vi "aFGV - Read Write Config.vi"(6 "State":enum16{"Read", "Write", "Delete"}(ring), 7 "Section":T1=enum."Calibration", 8 "Error In":errorcluster, 10 "Key Name":string, 11 "Data in":string[](array[string])) -> (0 "Error Out":errorcluster, 2 "Data out":string[](array[string]), 3 "Key Names":string[](array[string]))   [LabVIEW 2020]
uses:
  Control/Section.ctl
  Control/State - FGV.ctl
  <vilib>/Utility/config.llb/Read Key (String).vi
  <vilib>/Utility/config.llb/Write Key (String).vi
  <vilib>/Utility/config.llb/NI_LVConfig.lvlib
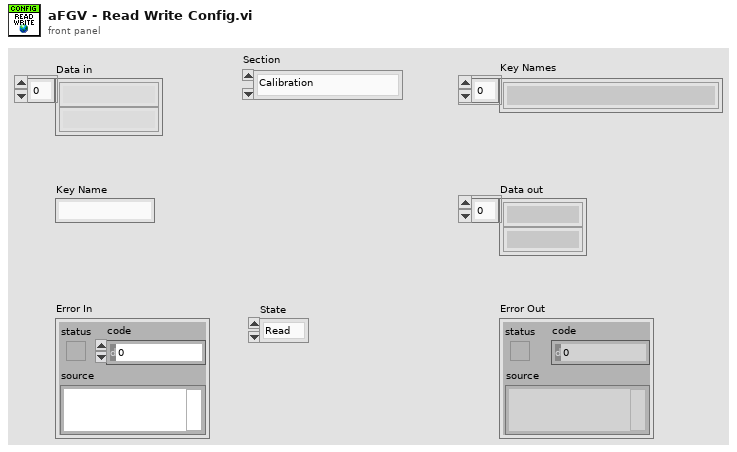
[diagram p1: front panel]
types:
  T1 = typedef "Section.ctl" = enum16{"Software Setup", "Config", "Setup", "Network Stream", "MQTT Client", "Setting", "Sample Interval", "Calibration", "Pre-Ranging", "Overrun", "Static", "Filter", "Properties", "Alarm", "Device", "Logging"}
  T2 = typedef "State - FGV.ctl" = enum16{"Write", "Read"}
  T3 = typedef "NI_LVConfig.lvlib/Config Data RefNum.ctl" = refnum<k1>
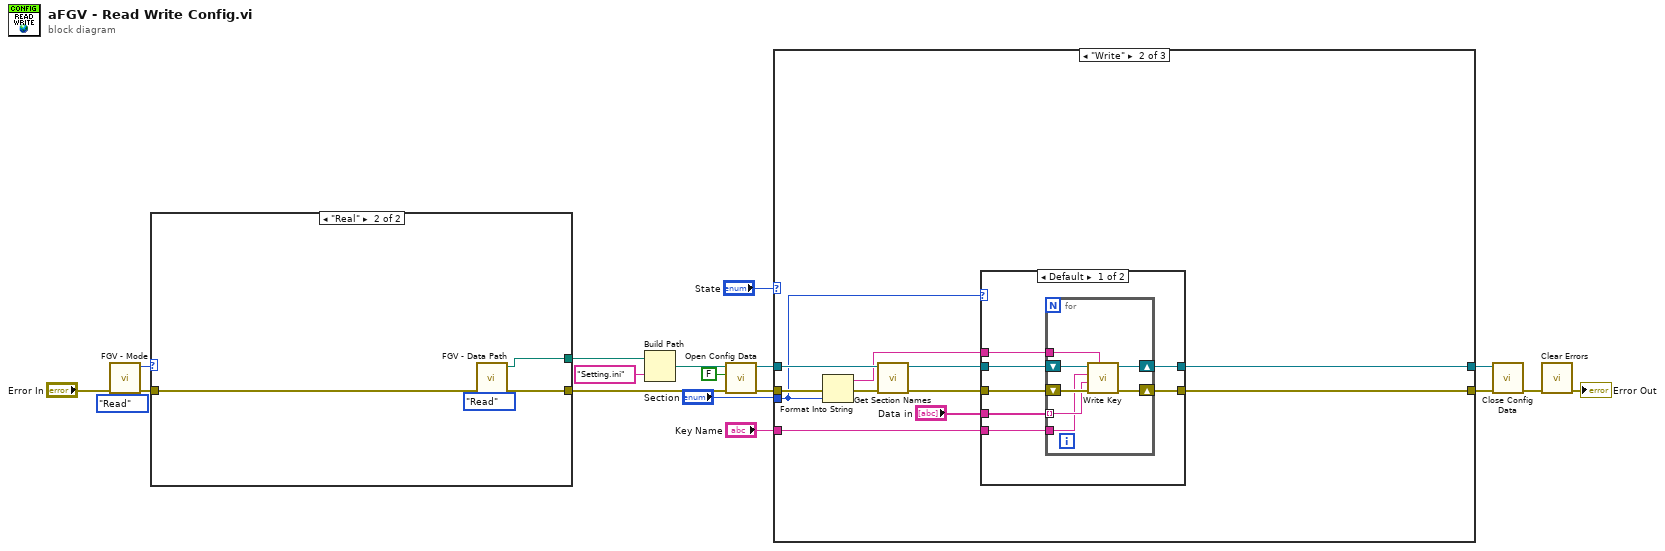
[diagram p0: block diagram]
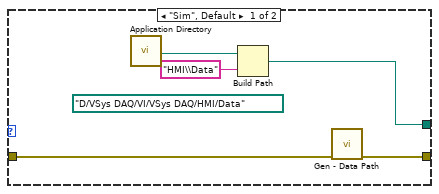
[diagram p2: hidden frame]
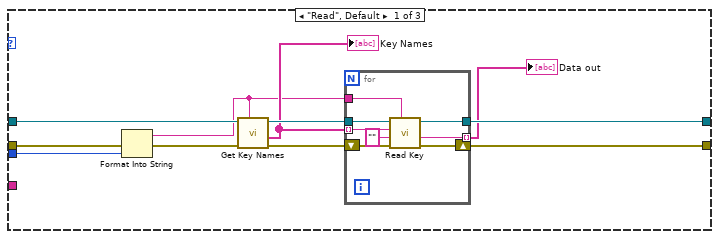
[diagram p3: hidden frame]
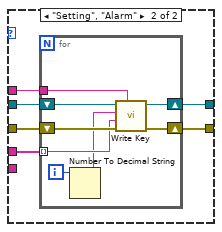
[diagram p4: hidden frame]
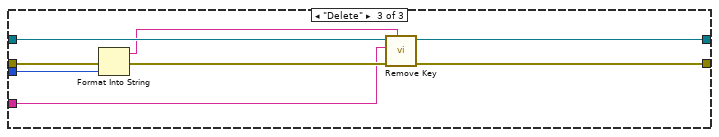
[diagram p5: hidden frame]
diagram:
  n1 = call "FGV - Mode.vi"("Action"=enum16{"Read", "Write"}."Read", "Error In"="Error In") -> ("Error Out"=w13:errorcluster, "Mode Out"=w3:enum16{"Sim", "Real"})  [unwired: 8 in]
  n2 = case shown="\"Real\"" w3 {
    tunnel: w13 -> [w23 w27]
    tunnel: [w22 w26] -> w12
    tunnel: [w19 w25] -> w2
    frame "Sim", Default {
      (unwired) path "D:/VSys DAQ/VI/VSys DAQ/HMI/Data" ("Path")
      n3 = call <vilib>:"Application Directory.vi"() -> ("Application Directory"=w21:path)
      n4 = Build Path(base path=w21, name or relative path="HMI\\Data") -> (appended path=w19:path)
      n5 = call "Gen - Data Path.vi"("Error In"=w23) -> ("Error Out"=w22:errorcluster)  [unwired: 9 in, 1 out]
    }
    frame "Real" {
      n6 = call "FGV - Data Path.vi"("FGV State"=State_-_FGV."Read", "Error In"=w27) -> ("Error Out"=w26:errorcluster, "Path Out"=w25:path)  [unwired: 8 in]
    }
  }
  n7 = Build Path(base path=w2, name or relative path="Setting.ini") -> (appended path=w8:path)
  n8 = call <vilib>:"Open Config Data.vi"("error in (no error)"=w12, "create file if necessary (T)"=FALSE, "configuration file path"=w8) -> ("error out"=w18:errorcluster, "refnum"=w11:T3)  [unwired: 6 in, 1 out]
  n9 = case shown="\"Write\"" "State" {
    tunnel: w18 -> [w35 w57 w93]
    tunnel: w11 -> [w34 w53 w90]
    tunnel: [w38 w56 w92] -> w17
    tunnel: [w33 w52 w88] -> w10
    tunnel: "Section" -> [w29 w48 w87]
    tunnel: "Key Name" -> [_ w49 w89]
    frame "Read", Default {
      n10 = Format Into String(error in=w35, w29) -> (resulting string=w28:string, error out=w36:errorcluster)  [unwired: 2 in]
      n11 = call <vilib>:"Get Key Names.vi"("section"=w28, "error in (no error)"=w36, "refnum"=w34) -> ("error out"=w37:errorcluster, "key names"=w31:string[], "refnum out"=w32:T3)  [unwired: 5 in, 1 out]
      "Key Names" <- w31
      n12 = for {
        tunnel: w32 -> [w44]
        shift-right: [w46] -> w38
        shift-left: w37 -> [w45]
        tunnel: w31 -> [w43] mode=indexing
        tunnel: w28 -> [w41]
        tunnel: [w40] -> w33
        tunnel: [w39] -> w30 mode=indexing
        n13 = call-poly <vilib>:"Read Key.vi"("section"=w41, "error in (no error)"=w45, "default value"="", "key"=w43, "refnum"=w44) -> ("error out"=w46:errorcluster, "value"=w39:string, "refnum out"=w40:T3)  [unwired: 3 in, 1 out]
      }
      "Data out" <- w30
    }
    frame "Write" {
      n14 = Format Into String(error in=w57, w48) -> (resulting string=w47:string, error out=w54:errorcluster)  [unwired: 2 in]
      n15 = call <vilib>:"Get Section Names.vi"("error in (no error)"=w54, "refnum"=w53) -> ("error out"=w55:errorcluster, "refnum out"=w51:T3)  [unwired: 7 in, 1 out]
      n16 = case shown="Default" w48 {
        tunnel: w55 -> [w64 w77]
        tunnel: [w63 w76] -> w56
        tunnel: w47 -> [w62 w75]
        tunnel: w51 -> [w61 w74]
        tunnel: [w60 w73] -> w52
        tunnel: "Data in" -> [w59 w72]
        tunnel: w49 -> [w58 _]
        frame Default {
          n17 = for {
            tunnel: w62 -> [w69]
            tunnel: w59 -> [w66] mode=indexing
            shift-right: [w70] -> w63
            shift-left: w64 -> [w71]
            shift-right: [w67] -> w60
            shift-left: w61 -> [w68]
            tunnel: w58 -> [w65]
            n18 = call-poly <vilib>:"Write Key.vi"("section"=w69, "error in (no error)"=w71, "value"=w66, "key"=w65, "refnum"=w68) -> ("error out"=w70:errorcluster, "refnum out"=w67:T3)  [unwired: 4 in, 1 out]
          }
        }
        frame "Setting", "Alarm" {
          n19 = for {
            tunnel: w75 -> [w83]
            tunnel: w72 -> [w80] mode=indexing
            shift-right: [w84] -> w76
            shift-left: w77 -> [w85]
            shift-right: [w81] -> w73
            shift-left: w74 -> [w82]
            i -> [w79]
            n20 = Number To Decimal String(number=w79) -> (decimal integer string=w78:string)  [unwired: 1 in]
            n21 = call-poly <vilib>:"Write Key.vi"("section"=w83, "error in (no error)"=w85, "value"=w80, "key"=w78, "refnum"=w82) -> ("error out"=w84:errorcluster, "refnum out"=w81:T3)  [unwired: 4 in, 1 out]
          }
        }
      }
    }
    frame "Delete" {
      n22 = Format Into String(error in=w93, w87) -> (resulting string=w86:string, error out=w91:errorcluster)  [unwired: 2 in]
      n23 = call <vilib>:"Remove Key.vi"("section"=w86, "error in (no error)"=w91, "key"=w89, "refnum"=w90) -> ("error out"=w92:errorcluster, "refnum out"=w88:T3)  [unwired: 5 in, 1 out]
    }
  }
  n24 = call <vilib>:"Close Config Data.vi"("error in (no error)"=w17, "refnum"=w10) -> ("error out"=w16:errorcluster)  [unwired: 8 in, 1 out]
  n25 = call <vilib>:"Clear Errors.vi"("error in (no error)"=w16) -> ("error out"=→"Error Out":errorcluster)  [unwired: 5 in, 1 out]
